vi "Puntos medios de pulso-inycom.vi"(8 "DI Inductivo":sgl[](array[numeric])) -> (0 "Puntos":sgl[](array[numeric]), 3 "Número de ejes":i32)   [LabVIEW 2015]
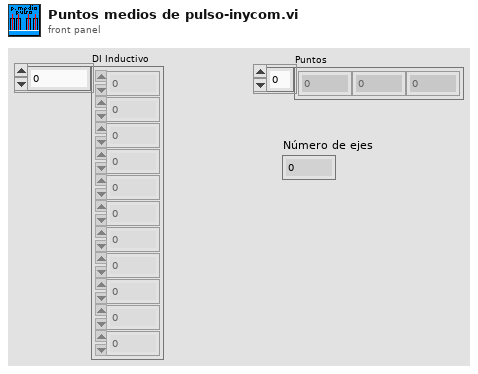
[diagram p1: front panel]
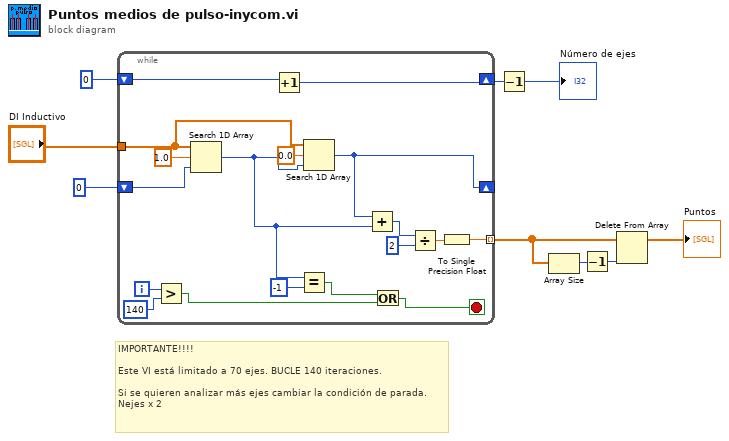
[diagram p0: block diagram]
diagram:
  # "IMPORTANTE!!!!\n\nEste VI está limitado a 70 ejes. BUCLE 140 iteraciones.\n\nSi se quieren analizar más ejes cambiar la condición de parada.\nNejes x 2"
  n1 = while {
    tunnel: "DI Inductivo" -> [w25]
    shift-right: [w19] -> _
    shift-left: 0 -> [w27]
    tunnel: [w20] -> w4 mode=indexing
    shift-right: [w15] -> w5
    shift-left: 0 -> [w16]
    i -> [w14]
    stop <- w10 stop-if-true
    n2 = Greater?(x=w14, y=140) -> (0:w11:bool)
    n3 = Search 1D Array(1D array=w25, element=sgl 1.0, start index (0)=w27) -> (index of element=w18:i32)
    n4 = Increment(x=w16) -> (x+1=w15:i32)
    n5 = Equal?(x=w18, y=-1) -> (x = y?=w12:bool)
    n6 = Search 1D Array(1D array=w25, element=sgl 0.0, start index (0)=w18) -> (index of element=w19:i32)
    n7 = Add(x=w19, y=w18) -> (x+y=w23:i32)
    n8 = Or(x=w12, y=w11) -> (x .or. y?=w10:bool)
    n9 = Divide(x=w23, y=2) -> (x/y=w21:dbl)
    n10 = To Single Precision Float(number=w21) -> (single precision float=w20:sgl)
  }
  n11 = Decrement(x=w5) -> (x-1=→"Número de ejes":i32)
  n12 = Array Size(array=w4) -> (size(s)=w3:i32)
  n13 = Decrement(x=w3) -> (x-1=w2:i32)
  n14 = Delete From Array(array=w4, index=w2) -> (array with subset deleted=→"Puntos":sgl[])  [unwired: 1 in, 1 out]
